vi "CRYResonance Curve.vi"(0 "Freq":dbl=100.0 format="%.2f", 1 "Low Freq":dbl=inf format="%.2f", 2 "Q":dbl=12.0 format="%.2f", 3 "Magn":dbl=1.0 format="%.2f", 4 "Resolution":dbl=80.0 min=0.0 max=160.0 step=10.0 format="%.2f", 5 "High Freq":dbl format="%.2f", 8 "Limit":dbl=0.5 min=0.0 max=1.0 step=0.1 format="%.2f") -> (7 "Output":cluster{"FStart":dbl, "Magn":dbl}[](array[cluster])=[{"FStart"=91.72759353897794, "Magn"=0.4341584458351582}, {"FStart"=94.40608762859233, "Magn"=0.5861305736585463}, {"FStart"=97.16279515771062, "Magn"=0.8227450296840774}, {"FStart"=100.0, "Magn"=1.0}, {"FStart"=102.92005271944282, "Magn"=0.8227450296840774}, {"FStart"=105.9253725177289, "Magn"=0.5861305736585453}, {"FStart"=109.01844923851279, "Magn"=0.4341584458351583}] {"Magn" format="%.2f"; "FStart" format="%.2f"})   [LabVIEW 2013]
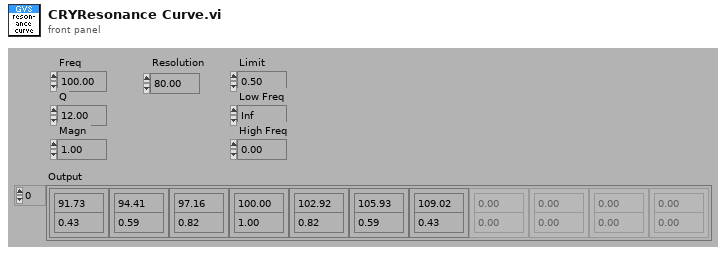
[diagram p1: front panel]
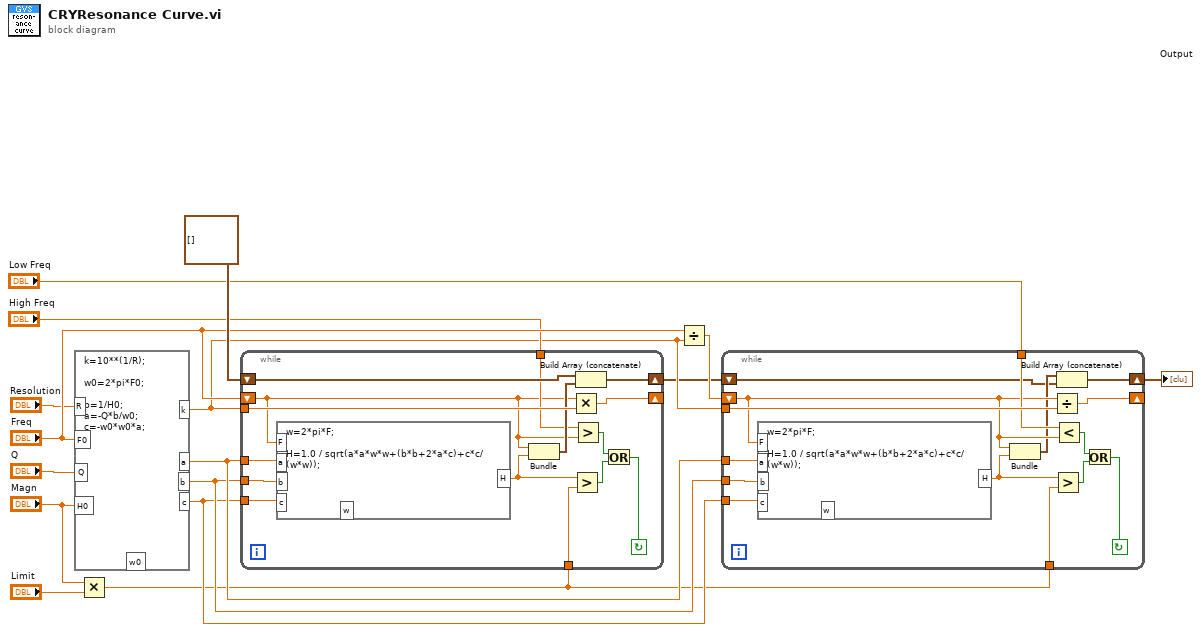
[diagram p0: block diagram]
diagram:
  n1 = formula code="k=10**(1/R);\n\nw0=2*pi*F0;\n\nb=1/H0;\na=-Q*b/w0;\nc=-w0*w0*a;"("F0"="Freq", "Q"="Q", "H0"="Magn", "R"="Resolution") -> ("a"=w7:dbl, "b"=w6:dbl, "c"=w5:dbl, "k"=w8:dbl)  [unwired: 1 out]
  n2 = Multiply(x="Magn", y="Limit") -> (x*y=w4:dbl)
  n3 = while {
    tunnel: "High Freq" -> [w21]
    tunnel: w4 -> [w22]
    shift-left: cluster{dbl, dbl}[] [] -> [w26]
    shift-right: [w24] -> w2
    tunnel: w5 -> [w27]
    tunnel: w6 -> [w28]
    tunnel: w7 -> [w29]
    tunnel: w8 -> [w31]
    shift-left: "Freq" -> [w20]
    shift-right: [w30] -> _
    stop <- w17 continue-if-true
    n4 = formula code="w=2*pi*F;\n\nH=1.0 / sqrt(a*a*w*w+(b*b+2*a*c)+c*c/(w*w));"("F"=w20, "a"=w29, "b"=w28, "c"=w27) -> ("H"=w23:dbl)  [unwired: 1 out]
    n5 = Bundle("Freq"=w20, "H"=w23) -> (w25:cluster{"Freq":dbl, "H":dbl})  [unwired: 1 out]
    n6 = Multiply(x=w20, y=w31) -> (x*y=w30:dbl)
    n7 = Greater?(x=w23, y=w22) -> (0:w18:bool)
    n8 = Greater?(x=w21, y=w20) -> (0:w19:bool)
    n9 = Build Array (concatenate)(w26, w25) -> (w24:cluster{"Freq":dbl, "H":dbl}[])
    n10 = Or(x=w19, y=w18) -> (x .or. y?=w17:bool)
  }
  n11 = Divide(x="Freq", y=w8) -> (x/y=w9:dbl)
  n12 = while {
    tunnel: "Low Freq" -> [w38]
    tunnel: w4 -> [w39]
    shift-left: w2 -> [w32]
    shift-right: [w41] -> w1
    tunnel: w5 -> [w42]
    tunnel: w6 -> [w43]
    tunnel: w7 -> [w44]
    tunnel: w8 -> [w46]
    shift-left: w9 -> [w37]
    shift-right: [w45] -> _
    stop <- w34 continue-if-true
    n13 = formula code="w=2*pi*F;\n\nH=1.0 / sqrt(a*a*w*w+(b*b+2*a*c)+c*c/(w*w));"("F"=w37, "a"=w44, "b"=w43, "c"=w42) -> ("H"=w40:dbl)  [unwired: 1 out]
    n14 = Bundle(w37, "H"=w40) -> (w33:cluster{dbl, "H":dbl})  [unwired: 1 out]
    n15 = Divide(x=w37, y=w46) -> (x/y=w45:dbl)
    n16 = Greater?(x=w40, y=w39) -> (0:w35:bool)
    n17 = Less?(x=w38, y=w37) -> (x < y?=w36:bool)
    n18 = Build Array (concatenate)(w33, w32) -> (w41:cluster{dbl, "H":dbl}[])
    n19 = Or(x=w36, y=w35) -> (x .or. y?=w34:bool)
  }
  "Output" <- w1
